vi "NI VeriStand - Close Macro Player Reference.vi"(8 "error in (no error)":errorcluster, 11 "MacroPlayer":T1) -> (0 "error out":errorcluster)   [LabVIEW 2020, in "NI_VS MacroPlayerAPI.lvlib"]
doc: "Closes an open reference to the Macro Player tool on the VeriStand Gateway. Use this VI to close each Macro Player reference that you open with the Open Macro Player Reference VI."
uses:
  <vilib>/NI VeriStand/Execution/MacroPlayer/NI_VS MacroPlayerAPI.lvlib
  <vilib>/NI VeriStand/Execution/MacroPlayer/MacroPlayerAPI.ctl
  NationalInstruments.VeriStand.ClientAPI
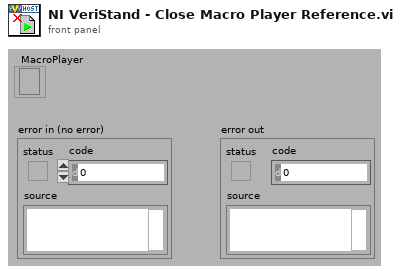
[diagram p1: front panel]
types:
  T1 = typedef "NI_VS MacroPlayerAPI.lvlib/MacroPlayerAPI.ctl" = refnum<k24>
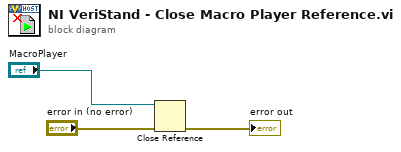
[diagram p0: block diagram]
diagram:
  n1 = Close Reference(reference="MacroPlayer", error in (no error)="error in (no error)") -> (error out=→"error out":errorcluster)
